vi "HFRR ADV v07.vi"() -> ()   [LabVIEW 2025] (continued)
            n1797 = local write "String 6"(w2052) -> ()
            n1798 = local write "String 7"(w2052) -> ()
            n1799 = local write "String 8"(w2052) -> ()
            n1800 = local write "String 12"(w2052) -> ()
            n1801 = local read "OK Button 16"() -> (w2037:bool)
            n1802 = String To Path(string=w2040) -> (path=w2048:path)
            n1803 = String To Path(string=w2039) -> (path=w2047:path)
            n1804 = String To Path(string=w2038) -> (path=w2046:path)
            n1805 = case shown="True" w2037 {
              tunnel: [w2053 w2054] -> w2041
              frame False {
                n1806 = local read "string1"() -> (w2053:string)
              }
              frame True {
                n1807 = local read "String Indicator 4"() -> (w2054:string)
              }
            }
            n1808 = Open/Create/Replace File "Open File"(file path (use dialog)=w2048) -> (refnum out=w2044:refnum<file>)  [unwired: 5 in, 2 out]
            n1809 = Open/Create/Replace File "Open File"(file path (use dialog)=w2047) -> (refnum out=w2043:refnum<file>)  [unwired: 5 in, 2 out]
            n1810 = Open/Create/Replace File "Open File"(file path (use dialog)=w2046) -> (refnum out=w2042:refnum<file>)  [unwired: 5 in, 2 out]
            n1811 = while {
              tunnel: w2044 -> [w2066]
              i -> [w2062]
              stop <- w2061 continue-if-true
              (unwired) TRUE ("line mode (F)")
              n1812 = Read from Text File "Read File"(file (use dialog)=w2066) -> (text=w2063:string)  [unwired: 3 in, 3 out]
              n1813 = local write "Numeric 11"(w2062) -> ()
              n1814 = String Length(string=w2063) -> (length=w2065:i32)
              n1815 = Greater?(x=w2065, y=1) -> (0:w2061:bool)
            }
            n1816 = while {
              tunnel: w2043 -> [w2072]
              i -> [w2068]
              stop <- w2067 continue-if-true
              (unwired) TRUE ("line mode (F)")
              n1817 = Read from Text File "Read File"(file (use dialog)=w2072) -> (text=w2069:string)  [unwired: 3 in, 3 out]
              n1818 = local write "Numeric 12"(w2068) -> ()
              n1819 = String Length(string=w2069) -> (length=w2071:i32)
              n1820 = Greater?(x=w2071, y=1) -> (0:w2067:bool)
            }
            n1821 = while {
              tunnel: w2042 -> [w2078]
              i -> [w2074]
              stop <- w2073 continue-if-true
              (unwired) TRUE ("line mode (F)")
              n1822 = Read from Text File "Read File"(file (use dialog)=w2078) -> (text=w2075:string)  [unwired: 3 in, 3 out]
              n1823 = local write "Numeric 13"(w2074) -> ()
              n1824 = String Length(string=w2075) -> (length=w2077:i32)
              n1825 = Greater?(x=w2077, y=1) -> (0:w2073:bool)
            }
            n1826 = String To Path(string=w2041) -> (path=w2049:path)
            n1827 = Open/Create/Replace File "Open File"(file path (use dialog)=w2049) -> (refnum out=w2045:refnum<file>)  [unwired: 5 in, 2 out]
            n1828 = while {
              tunnel: w2045 -> [w2060]
              i -> [w2056]
              stop <- w2055 continue-if-true
              (unwired) TRUE ("line mode (F)")
              n1829 = Read from Text File "Read File"(file (use dialog)=w2060) -> (text=w2057:string)  [unwired: 3 in, 3 out]
              n1830 = local write "Numeric 8"(w2056) -> ()
              n1831 = String Length(string=w2057) -> (length=w2059:i32)
              n1832 = Greater?(x=w2059, y=1) -> (0:w2055:bool)
            }
          }
          frame #1 {
            w2230 = FALSE ("ACTUAL   MERGE")
            # "Sample Temp"
            # "ECR"
            # "COF"
            # "Time\nCOF\nFF\nTemp"
            n1833 = case shown="True" w2103 {
              tunnel: [w2250 w2251] -> w2104
              frame False {
                n1834 = local read "string1"() -> (w2250:string)
              }
              frame True {
                n1835 = local read "String Indicator 4"() -> (w2251:string)
              }
            }
            n1836 = local read "string1 3"() -> (w2148:string)
            n1837 = String To Path(string=w2104) -> (path=w2235:path)
            n1838 = String To Path(string=w2148) -> (path=w2246:path)
            n1839 = local read "Numeric 12"() -> (w2232:i32)
            n1840 = local read "Numeric 8"() -> (w2234:i32)
            n1841 = local read "string1 2"() -> (w2149:string)
            n1842 = local read "string1 4"() -> (w2147:string)
            n1843 = Open/Create/Replace File "Open File"(file path (use dialog)=w2235) -> (refnum out=w2249:refnum<file>, error out=w2248:errorcluster)  [unwired: 5 in, 1 out]
            n1844 = Open/Create/Replace File "Open File"(file path (use dialog)=w2246) -> (refnum out=w2242:refnum<file>, error out=w2243:errorcluster)  [unwired: 5 in, 1 out]
            n1845 = for {
              N: w2234 -> [_]
              tunnel: w2249 -> [w2397]
              tunnel: w2248 -> [w2396]
              tunnel: [w2386] -> w2161 mode=indexing
              tunnel: [w2384] -> w2218 mode=indexing
              tunnel: [w2385] -> w2213 mode=indexing
              tunnel: w2230 -> [_]
              tunnel: [w2378] -> w2215 mode=indexing
              tunnel: [w2374] -> w2184 mode=indexing
              tunnel: [w2370] -> w2159 mode=indexing
              tunnel: [w2366] -> w2140 mode=indexing
              tunnel: [w2361] -> w2100 mode=indexing
              (unwired) TRUE ("line mode (F)")
              # "freq"
              # "Stroke"
              # "Time"
              # "CoF"
              # "Humidity"
              # "Temp"
              # "Air Temp"
              # "ECR"
              n1846 = Read from Text File "Read File"(file (use dialog)=w2397, error in=w2396) -> (text=w2362:string)  [unwired: 2 in, 3 out]
              n1847 = local write "String 6"(w2362) -> ()
              n1848 = String Subset(string=w2362, offset (0)=0, length (rest)=14 ("length (rest)")) -> (substring=w2390:string)
              n1849 = String Subset(string=w2362, offset (0)=35, length (rest)=9 ("length (rest)")) -> (substring=w2387:string)
              n1850 = String Subset(string=w2362, offset (0)=15, length (rest)=9 ("length (rest)")) -> (substring=w2393:string)
              n1851 = Fract/Exp String To Number(string=w2390) -> (number=w2386:dbl)  [unwired: 3 in, 1 out]
              n1852 = Fract/Exp String To Number(string=w2387) -> (number=w2385:dbl)  [unwired: 3 in, 1 out]
              n1853 = Fract/Exp String To Number(string=w2393) -> (number=w2384:dbl)  [unwired: 3 in, 1 out]
              n1854 = String Subset(string=w2362, offset (0)=85, length (rest)=9 ("length (rest)")) -> (substring=w2363:string)
              n1855 = String Subset(string=w2362, offset (0)=25, length (rest)=9 ("length (rest)")) -> (substring=w2369:string)
              n1856 = String Subset(string=w2362, offset (0)=55, length (rest)=9 ("length (rest)")) -> (substring=w2371:string)
              n1857 = String Subset(string=w2362, offset (0)=45, length (rest)=9 ("length (rest)")) -> (substring=w2377:string)
              n1858 = String Subset(string=w2362, offset (0)=65, length (rest)=9 ("length (rest)")) -> (substring=w2383:string)
              n1859 = Fract/Exp String To Number(string=w2369) -> (number=w2366:dbl)  [unwired: 3 in, 1 out]
              n1860 = Fract/Exp String To Number(string=w2363) -> (number=w2361:dbl)  [unwired: 3 in, 1 out]
              n1861 = Fract/Exp String To Number(string=w2371) -> (number=w2370:dbl)  [unwired: 3 in, 1 out]
              n1862 = Fract/Exp String To Number(string=w2377) -> (number=w2374:dbl)  [unwired: 3 in, 1 out]
              n1863 = Fract/Exp String To Number(string=w2383) -> (number=w2380:dbl)  [unwired: 3 in, 1 out]
              n1864 = Add(x=w2380, y=0.0) -> (x+y=w2378:dbl)
            }
            n1865 = for {
              N: w2232 -> [_]
              tunnel: w2243 -> [w2323]
              tunnel: w2242 -> [w2322]
              tunnel: [w2312] -> w2201 mode=indexing
              tunnel: [w2310] -> w2199 mode=indexing
              tunnel: [w2311] -> w2195 mode=indexing
              tunnel: w2230 -> [_]
              tunnel: [w2304] -> w2197 mode=indexing
              tunnel: [w2300] -> w2179 mode=indexing
              tunnel: [w2296] -> w2155 mode=indexing
              tunnel: [w2293] -> w2136 mode=indexing
              tunnel: [w2289] -> w2095 mode=indexing
              (unwired) 9 ("length (rest)")
              (unwired) 9 ("length (rest)")
              (unwired) TRUE ("line mode (F)")
              n1866 = Read from Text File "Read File"(file (use dialog)=w2322, error in=w2323) -> (text=w2290:string)  [unwired: 2 in, 3 out]
              n1867 = local write "String 8"(w2290) -> ()
              n1868 = String Subset(string=w2290, offset (0)=85) -> (substring=w2292:string)  [unwired: 1 in]
              n1869 = String Subset(string=w2290, offset (0)=35, length (rest)=9 ("length (rest)")) -> (substring=w2313:string)
              n1870 = String Subset(string=w2290, offset (0)=55, length (rest)=9 ("length (rest)")) -> (substring=w2298:string)
              n1871 = String Subset(string=w2290, offset (0)=25) -> (substring=w2294:string)  [unwired: 1 in]
              n1872 = String Subset(string=w2290, offset (0)=15, length (rest)=9 ("length (rest)")) -> (substring=w2319:string)
              n1873 = String Subset(string=w2290, offset (0)=0, length (rest)=14 ("length (rest)")) -> (substring=w2316:string)
              n1874 = String Subset(string=w2290, offset (0)=45, length (rest)=9 ("length (rest)")) -> (substring=w2303:string)
              n1875 = String Subset(string=w2290, offset (0)=65, length (rest)=9 ("length (rest)")) -> (substring=w2309:string)
              n1876 = Fract/Exp String To Number(string=w2292) -> (number=w2289:dbl)  [unwired: 3 in, 1 out]
              n1877 = Fract/Exp String To Number(string=w2313) -> (number=w2311:dbl)  [unwired: 3 in, 1 out]
              n1878 = Fract/Exp String To Number(string=w2298) -> (number=w2296:dbl)  [unwired: 3 in, 1 out]
              n1879 = Fract/Exp String To Number(string=w2294) -> (number=w2293:dbl)  [unwired: 3 in, 1 out]
              n1880 = Fract/Exp String To Number(string=w2319) -> (number=w2310:dbl)  [unwired: 3 in, 1 out]
              n1881 = Fract/Exp String To Number(string=w2316) -> (number=w2312:dbl)  [unwired: 3 in, 1 out]
              n1882 = Fract/Exp String To Number(string=w2303) -> (number=w2300:dbl)  [unwired: 3 in, 1 out]
              n1883 = Fract/Exp String To Number(string=w2309) -> (number=w2306:dbl)  [unwired: 3 in, 1 out]
              n1884 = Add(x=w2306, y=0.0) -> (x+y=w2304:dbl)
            }
            n1885 = String To Path(string=w2149) -> (path=w2247:path)
            n1886 = String To Path(string=w2147) -> (path=w2241:path)
            n1887 = local read "Numeric 11"() -> (w2231:i32)
            n1888 = local read "Numeric 13"() -> (w2233:i32)
            n1889 = Open/Create/Replace File "Open File"(file path (use dialog)=w2247) -> (refnum out=w2245:refnum<file>, error out=w2244:errorcluster)  [unwired: 5 in, 1 out]
            n1890 = Open/Create/Replace File "Open File"(file path (use dialog)=w2241) -> (refnum out=w2240:refnum<file>, error out=w2239:errorcluster)  [unwired: 5 in, 1 out]
            n1891 = for {
              N: w2231 -> [_]
              tunnel: w2245 -> [w2360]
              tunnel: w2244 -> [w2359]
              tunnel: [w2349] -> w2211 mode=indexing
              tunnel: [w2347] -> w2209 mode=indexing
              tunnel: [w2348] -> w2204 mode=indexing
              tunnel: w2230 -> [_]
              tunnel: [w2341] -> w2206 mode=indexing
              tunnel: [w2337] -> w2182 mode=indexing
              tunnel: [w2333] -> w2157 mode=indexing
              tunnel: [w2329] -> w2138 mode=indexing
              tunnel: [w2324] -> w2096 mode=indexing
              (unwired) TRUE ("line mode (F)")
              n1892 = Read from Text File "Read File"(file (use dialog)=w2360, error in=w2359) -> (text=w2325:string)  [unwired: 2 in, 3 out]
              n1893 = local write "String 7"(w2325) -> ()
              n1894 = String Subset(string=w2325, offset (0)=85, length (rest)=9 ("length (rest)")) -> (substring=w2328:string)
              n1895 = String Subset(string=w2325, offset (0)=35, length (rest)=9 ("length (rest)")) -> (substring=w2350:string)
              n1896 = String Subset(string=w2325, offset (0)=55, length (rest)=9 ("length (rest)")) -> (substring=w2336:string)
              n1897 = String Subset(string=w2325, offset (0)=25, length (rest)=9 ("length (rest)")) -> (substring=w2330:string)
              n1898 = String Subset(string=w2325, offset (0)=45, length (rest)=9 ("length (rest)")) -> (substring=w2338:string)
              n1899 = String Subset(string=w2325, offset (0)=0, length (rest)=14 ("length (rest)")) -> (substring=w2353:string)
              n1900 = String Subset(string=w2325, offset (0)=15, length (rest)=9 ("length (rest)")) -> (substring=w2356:string)
              n1901 = String Subset(string=w2325, offset (0)=65, length (rest)=9 ("length (rest)")) -> (substring=w2342:string)
              n1902 = Fract/Exp String To Number(string=w2328) -> (number=w2324:dbl)  [unwired: 3 in, 1 out]
              n1903 = Fract/Exp String To Number(string=w2350) -> (number=w2348:dbl)  [unwired: 3 in, 1 out]
              n1904 = Fract/Exp String To Number(string=w2336) -> (number=w2333:dbl)  [unwired: 3 in, 1 out]
              n1905 = Fract/Exp String To Number(string=w2330) -> (number=w2329:dbl)  [unwired: 3 in, 1 out]
              n1906 = Fract/Exp String To Number(string=w2338) -> (number=w2337:dbl)  [unwired: 3 in, 1 out]
              n1907 = Fract/Exp String To Number(string=w2353) -> (number=w2349:dbl)  [unwired: 3 in, 1 out]
              n1908 = Fract/Exp String To Number(string=w2356) -> (number=w2347:dbl)  [unwired: 3 in, 1 out]
              n1909 = Fract/Exp String To Number(string=w2342) -> (number=w2345:dbl)  [unwired: 3 in, 1 out]
              n1910 = Add(x=w2345, y=0.0) -> (x+y=w2341:dbl)
            }
            n1911 = for {
              N: w2233 -> [_]
              tunnel: w2240 -> [w2288]
              tunnel: w2239 -> [w2287]
              tunnel: [w2277] -> w2193 mode=indexing
              tunnel: [w2276] -> w2186 mode=indexing
              tunnel: w2230 -> [_]
              tunnel: [w2265] -> w2191 mode=indexing
              tunnel: [w2270] -> w2188 mode=indexing
              tunnel: [w2266] -> w2178 mode=indexing
              tunnel: [w2261] -> w2153 mode=indexing
              tunnel: [w2257] -> w2134 mode=indexing
              tunnel: [w2252] -> w2094 mode=indexing
              (unwired) 1.0 ("x")
              (unwired) TRUE ("line mode (F)")
              n1912 = Read from Text File "Read File"(file (use dialog)=w2288, error in=w2287) -> (text=w2253:string)  [unwired: 2 in, 3 out]
              n1913 = local write "String 12"(w2253) -> ()
              n1914 = String Subset(string=w2253, offset (0)=85, length (rest)=9 ("length (rest)")) -> (substring=w2255:string)
              n1915 = String Subset(string=w2253, offset (0)=35, length (rest)=9 ("length (rest)")) -> (substring=w2278:string)
              n1916 = String Subset(string=w2253, offset (0)=55, length (rest)=9 ("length (rest)")) -> (substring=w2263:string)
              n1917 = String Subset(string=w2253, offset (0)=25, length (rest)=9 ("length (rest)")) -> (substring=w2259:string)
              n1918 = String Subset(string=w2253, offset (0)=45, length (rest)=9 ("length (rest)")) -> (substring=w2268:string)
              n1919 = String Subset(string=w2253, offset (0)=15, length (rest)=9 ("length (rest)")) -> (substring=w2284:string)
              n1920 = String Subset(string=w2253, offset (0)=0, length (rest)=14 ("length (rest)")) -> (substring=w2281:string)
              n1921 = String Subset(string=w2253, offset (0)=65, length (rest)=9 ("length (rest)")) -> (substring=w2271:string)
              n1922 = Fract/Exp String To Number(string=w2255) -> (number=w2252:dbl)  [unwired: 3 in, 1 out]
              n1923 = Fract/Exp String To Number(string=w2278) -> (number=w2276:dbl)  [unwired: 3 in, 1 out]
              n1924 = Fract/Exp String To Number(string=w2263) -> (number=w2261:dbl)  [unwired: 3 in, 1 out]
              n1925 = Fract/Exp String To Number(string=w2259) -> (number=w2257:dbl)  [unwired: 3 in, 1 out]
              n1926 = Fract/Exp String To Number(string=w2268) -> (number=w2266:dbl)  [unwired: 3 in, 1 out]
              n1927 = Fract/Exp String To Number(string=w2284) -> (number=w2265:dbl)  [unwired: 3 in, 1 out]
              n1928 = Fract/Exp String To Number(string=w2281) -> (number=w2277:dbl)  [unwired: 3 in, 1 out]
              n1929 = Fract/Exp String To Number(string=w2271) -> (number=w2274:dbl)  [unwired: 3 in, 1 out]
              n1930 = Add(x=w2274, y=0.0) -> (x+y=w2270:dbl)
            }
            n1931 = Delete From Array(array=w2136, index=0) -> (array with subset deleted=w2109:dbl[])  [unwired: 1 in, 1 out]
            n1932 = Delete From Array(array=w2199, index=0) -> (array with subset deleted=w2172:dbl[])  [unwired: 1 in, 1 out]
            n1933 = Delete From Array(array=w2179, index=0) -> (array with subset deleted=w2167:dbl[])  [unwired: 1 in, 1 out]
            n1934 = Delete From Array(array=w2197, index=0) -> (array with subset deleted=w2198:dbl[])  [unwired: 1 in, 1 out]
            n1935 = call-poly <vilib>:"Mean.vi"("X"=w2109) -> ("mean"=→"КОФ2 4":dbl)  [unwired: 1 out]
            n1936 = call-poly <vilib>:"Mean.vi"("X"=w2172) -> ("mean"=→"КОФ3":dbl)  [unwired: 1 out]
            n1937 = call-poly <vilib>:"Mean.vi"("X"=w2167) -> ("mean"=→"CP3":dbl)  [unwired: 1 out]
            n1938 = Delete From Array(array=w2161, index=0) -> (array with subset deleted=w2088:dbl[])  [unwired: 1 in, 1 out]
            n1939 = Delete From Array(array=w2100, index=0) -> (array with subset deleted=w2087:dbl[])  [unwired: 1 in, 1 out]
            n1940 = Delete From Array(array=w2140, index=0) -> (array with subset deleted=w2111:dbl[])  [unwired: 1 in, 1 out]
            n1941 = Delete From Array(array=w2218, index=0) -> (array with subset deleted=w2173:dbl[])  [unwired: 1 in, 1 out]
            n1942 = Delete From Array(array=w2184, index=0) -> (array with subset deleted=w2169:dbl[])  [unwired: 1 in, 1 out]
            "array w/ subset deleted" <- w2169
            n1943 = Delete From Array(array=w2215, index=0) -> (array with subset deleted=w2216:dbl[])  [unwired: 1 in, 1 out]
            n1944 = call-poly <vilib>:"Mean.vi"("X"=w2111) -> ("mean"=→"КОФ2 2":dbl)  [unwired: 1 out]
            n1945 = call-poly <vilib>:"Mean.vi"("X"=w2173) -> ("mean"=→"КОФ1":dbl)  [unwired: 1 out]
            n1946 = Bundle "Bundle"(w2088, w2087) -> (w2093:cluster{dbl[], dbl[]})  [unwired: 1 in]
            n1947 = Bundle "Bundle"(w2088, w2216) -> (w2080:cluster{dbl[], dbl[]})  [unwired: 1 in]
            n1948 = Delete From Array(array=w2095, index=0) -> (array with subset deleted=w2083:dbl[])  [unwired: 1 in, 1 out]
            n1949 = Delete From Array(array=w2096, index=0) -> (array with subset deleted=w2085:dbl[])  [unwired: 1 in, 1 out]
            n1950 = Delete From Array(array=w2206, index=0) -> (array with subset deleted=w2207:dbl[])  [unwired: 1 in, 1 out]
            n1951 = Delete From Array(array=w2094, index=0) -> (array with subset deleted=w2081:dbl[])  [unwired: 1 in, 1 out]
            n1952 = Delete From Array(array=w2188, index=0) -> (array with subset deleted=w2189:dbl[])  [unwired: 1 in, 1 out]
            n1953 = Delete From Array(array=w2213, index=0) -> (array with subset deleted=w2119:dbl[])  [unwired: 1 in, 1 out]
            n1954 = Delete From Array(array=w2159, index=0) -> (array with subset deleted=w2115:dbl[])  [unwired: 1 in, 1 out]
            n1955 = Delete From Array(array=w2195, index=0) -> (array with subset deleted=w2117:dbl[])  [unwired: 1 in, 1 out]
            n1956 = Delete From Array(array=w2155, index=0) -> (array with subset deleted=w2113:dbl[])  [unwired: 1 in, 1 out]
            n1957 = Delete From Array(array=w2204, index=0) -> (array with subset deleted=w2118:dbl[])  [unwired: 1 in, 1 out]
            n1958 = Delete From Array(array=w2157, index=0) -> (array with subset deleted=w2114:dbl[])  [unwired: 1 in, 1 out]
            n1959 = Delete From Array(array=w2138, index=0) -> (array with subset deleted=w2110:dbl[])  [unwired: 1 in, 1 out]
            n1960 = Delete From Array(array=w2182, index=0) -> (array with subset deleted=w2168:dbl[])  [unwired: 1 in, 1 out]
            n1961 = Delete From Array(array=w2209, index=0) -> (array with subset deleted=w2170:dbl[])  [unwired: 1 in, 1 out]
            n1962 = Delete From Array(array=w2186, index=0) -> (array with subset deleted=w2116:dbl[])  [unwired: 1 in, 1 out]
            n1963 = Delete From Array(array=w2153, index=0) -> (array with subset deleted=w2112:dbl[])  [unwired: 1 in, 1 out]
            n1964 = Delete From Array(array=w2134, index=0) -> (array with subset deleted=w2108:dbl[])  [unwired: 1 in, 1 out]
            n1965 = Delete From Array(array=w2178, index=0) -> (array with subset deleted=w2166:dbl[])  [unwired: 1 in, 1 out]
            n1966 = Delete From Array(array=w2191, index=0) -> (array with subset deleted=w2171:dbl[])  [unwired: 1 in, 1 out]
            n1967 = Delete From Array(array=w2201, index=0) -> (array with subset deleted=w2084:dbl[])  [unwired: 1 in, 1 out]
            n1968 = Delete From Array(array=w2211, index=0) -> (array with subset deleted=w2086:dbl[])  [unwired: 1 in, 1 out]
            n1969 = Delete From Array(array=w2193, index=0) -> (array with subset deleted=w2082:dbl[])  [unwired: 1 in, 1 out]
            n1970 = Bundle "Bundle"(w2088, w2119) -> (w2106:cluster{dbl[], dbl[]})  [unwired: 1 in]
            n1971 = Bundle "Bundle"(w2088, w2173) -> (w2107:cluster{dbl[], dbl[]})  [unwired: 1 in]
            n1972 = Bundle "Bundle"(w2119, w2115) -> (w2121:cluster{dbl[], dbl[]})  [unwired: 1 in]
            n1973 = Bundle "Bundle"(w2084, w2083) -> (w2091:cluster{dbl[], dbl[]})  [unwired: 1 in]
            n1974 = Bundle "Bundle"(w2117, w2113) -> (w2123:cluster{dbl[], dbl[]})  [unwired: 1 in]
            n1975 = Bundle "Bundle"(w2084, w2117) -> (w2227:cluster{dbl[], dbl[]})  [unwired: 1 in]
            n1976 = Bundle "Bundle"(w2084, w2113) -> (w2151:cluster{dbl[], dbl[]})  [unwired: 1 in]
            n1977 = Bundle "Bundle"(w2084, w2172) -> (w2237:cluster{dbl[], dbl[]})  [unwired: 1 in]
            n1978 = Bundle "Bundle"(w2084, w2167) -> (w2175:cluster{dbl[], dbl[]})  [unwired: 1 in]
            n1979 = Bundle "Bundle"(w2084, w2198) -> (w2222:cluster{dbl[], dbl[]})  [unwired: 1 in]
            n1980 = Bundle "Bundle"(w2118, w2114) -> (w2122:cluster{dbl[], dbl[]})  [unwired: 1 in]
            n1981 = Bundle "Bundle"(w2086, w2085) -> (w2092:cluster{dbl[], dbl[]})  [unwired: 1 in]
            n1982 = Bundle "Bundle"(w2086, w2118) -> (w2229:cluster{dbl[], dbl[]})  [unwired: 1 in]
            n1983 = Bundle "Bundle"(w2086, w2114) -> (w2152:cluster{dbl[], dbl[]})  [unwired: 1 in]
            n1984 = Bundle "Bundle"(w2086, w2168) -> (w2176:cluster{dbl[], dbl[]})  [unwired: 1 in]
            n1985 = Bundle "Bundle"(w2086, w2170) -> (w2238:cluster{dbl[], dbl[]})  [unwired: 1 in]
            n1986 = Bundle "Bundle"(w2086, w2207) -> (w2220:cluster{dbl[], dbl[]})  [unwired: 1 in]
            n1987 = Bundle "Bundle"(w2116, w2112) -> (w2124:cluster{dbl[], dbl[]})  [unwired: 1 in]
            n1988 = Bundle "Bundle"(w2082, w2081) -> (w2090:cluster{dbl[], dbl[]})  [unwired: 1 in]
            n1989 = Bundle "Bundle"(w2082, w2116) -> (w2228:cluster{dbl[], dbl[]})  [unwired: 1 in]
            n1990 = Bundle "Bundle"(w2082, w2112) -> (w2150:cluster{dbl[], dbl[]})  [unwired: 1 in]
            n1991 = Bundle "Bundle"(w2082, w2166) -> (w2174:cluster{dbl[], dbl[]})  [unwired: 1 in]
            n1992 = Bundle "Bundle"(w2082, w2171) -> (w2236:cluster{dbl[], dbl[]})  [unwired: 1 in]
            n1993 = Bundle "Bundle"(w2082, w2189) -> (w2221:cluster{dbl[], dbl[]})  [unwired: 1 in]
            n1994 = call-poly <vilib>:"Mean.vi"("X"=w2169) -> ("mean"=→"CP1":dbl)  [unwired: 1 out]
            n1995 = call-poly <vilib>:"Mean.vi"("X"=w2110) -> ("mean"=→"КОФ2 3":dbl)  [unwired: 1 out]
            n1996 = call-poly <vilib>:"Mean.vi"("X"=w2168) -> ("mean"=→"CP2":dbl)  [unwired: 1 out]
            n1997 = call-poly <vilib>:"Mean.vi"("X"=w2170) -> ("mean"=→"КОФ2":dbl)  [unwired: 1 out]
            n1998 = call-poly <vilib>:"Mean.vi"("X"=w2108) -> ("mean"=→"КОФ2 5":dbl)  [unwired: 1 out]
            n1999 = call-poly <vilib>:"Mean.vi"("X"=w2166) -> ("mean"=→"CP4":dbl)  [unwired: 1 out]
            n2000 = call-poly <vilib>:"Mean.vi"("X"=w2171) -> ("mean"=→"КОФ4":dbl)  [unwired: 1 out]
            n2001 = Bundle "Bundle"(w2088, w2115) -> (w2079:cluster{dbl[], dbl[]})  [unwired: 1 in]
            n2002 = Bundle "Bundle"(w2088, w2169) -> (w2102:cluster{dbl[], dbl[]})  [unwired: 1 in]
            n2003 = Build Array "Build Array"(w2079, w2102) -> (w2105:cluster{dbl[], dbl[]}[])
            "XY Graph 17" <- w2105
            n2004 = Build Array "Build Array"(w2093, w2092, w2091, w2090) -> (→"Frequency ( Hz )":cluster{dbl[], dbl[]}[])
            n2005 = Build Array "Build Array"(w2121, w2122, w2123, w2124) -> (→"Air Temp ( °C ) vs Humidity ( % RH )":cluster{dbl[], dbl[]}[])
            n2006 = Build Array "Build Array"(w2106, w2229, w2227, w2228) -> (→"Air Temperature  ( °C )":cluster{dbl[], dbl[]}[])
            n2007 = Build Array "Build Array"(w2079, w2152, w2151, w2150) -> (→"Humidity ( %RH )":cluster{dbl[], dbl[]}[])
            n2008 = Build Array "Build Array"(w2107, w2238, w2237, w2236) -> (→"Coefficient Of Friction":cluster{dbl[], dbl[]}[])
            n2009 = Build Array "Build Array"(w2102, w2176, w2175, w2174) -> (→"Sample Temperature ( °C )":cluster{dbl[], dbl[]}[])
            n2010 = Build Array "Build Array"(w2080, w2220, w2222, w2221) -> (→"XY Graph 13":cluster{dbl[], dbl[]}[])
            n2011 = Bundle "Bundle"(w2088, w2111) -> (w2133:cluster{dbl[], dbl[]})  [unwired: 1 in]
            n2012 = Bundle "Bundle"(w2084, w2109) -> (w2131:cluster{dbl[], dbl[]})  [unwired: 1 in]
            n2013 = Bundle "Bundle"(w2086, w2110) -> (w2132:cluster{dbl[], dbl[]})  [unwired: 1 in]
            n2014 = Bundle "Bundle"(w2082, w2108) -> (w2130:cluster{dbl[], dbl[]})  [unwired: 1 in]
            n2015 = Build Array "Build Array"(w2133, w2132, w2131, w2130) -> (→"Stroke ( mm )":cluster{dbl[], dbl[]}[])
            n2016 = local write "XY Graph 16"(w2105) -> ()
          }
          frame #2 {
          }
          frame #3 {
            n2017 = local write "Numeric 8"(0 ("Numeric 8")) -> ()
            n2018 = local write "Numeric 11"(0 ("Numeric 11")) -> ()
            n2019 = local write "Numeric 12"(0 ("Numeric 12")) -> ()
            n2020 = local write "Numeric 13"(0 ("Numeric 13")) -> ()
            n2021 = property on="OPEN" class="Bool (strict)"("Visible"=TRUE) -> ()  [unwired: 2 in, 2 out]
            n2022 = local read "String Control 2"() -> (w2405:string)
            n2023 = local read "String Control 4"() -> (w2404:string)
            n2024 = local read "String Control 6"() -> (w2403:string)
            n2025 = local read "String Control 8"() -> (w2402:string)
            n2026 = Match Pattern(string=w2405, regular expression="Samples / cycle :- ") -> (after substring=w2419:string)  [unwired: 1 in, 3 out]
            n2027 = Match Pattern(string=w2405, regular expression="Frequency :- ") -> (after substring=w2438:string)  [unwired: 1 in, 3 out]
            n2028 = Match Pattern(string=w2404, regular expression="Samples / cycle :- ") -> (after substring=w2415:string)  [unwired: 1 in, 3 out]
            n2029 = Match Pattern(string=w2404, regular expression="Frequency :- ") -> (after substring=w2433:string)  [unwired: 1 in, 3 out]
            n2030 = Match Pattern(string=w2403, regular expression="Samples / cycle :- ") -> (after substring=w2411:string)  [unwired: 1 in, 3 out]
            n2031 = Match Pattern(string=w2403, regular expression="Frequency :- ") -> (after substring=w2428:string)  [unwired: 1 in, 3 out]
            n2032 = Match Pattern(string=w2402, regular expression="Samples / cycle :- ") -> (after substring=w2407:string)  [unwired: 1 in, 3 out]
            n2033 = Match Pattern(string=w2402, regular expression="Frequency :- ") -> (after substring=w2423:string)  [unwired: 1 in, 3 out]
            n2034 = String Subset(string=w2419, length (rest)=6 ("length (rest)")) -> (substring=w2421:string)  [unwired: 1 in]
            n2035 = String Subset(string=w2438, length (rest)=9 ("length (rest)")) -> (substring=w2440:string)  [unwired: 1 in]
            n2036 = String Subset(string=w2415, length (rest)=6 ("length (rest)")) -> (substring=w2417:string)  [unwired: 1 in]
            n2037 = String Subset(string=w2433, length (rest)=9 ("length (rest)")) -> (substring=w2435:string)  [unwired: 1 in]
            n2038 = String Subset(string=w2411, length (rest)=6 ("length (rest)")) -> (substring=w2413:string)  [unwired: 1 in]
            n2039 = String Subset(string=w2428, length (rest)=9 ("length (rest)")) -> (substring=w2430:string)  [unwired: 1 in]
            n2040 = String Subset(string=w2407, length (rest)=6 ("length (rest)")) -> (substring=w2409:string)  [unwired: 1 in]
            n2041 = String Subset(string=w2423, length (rest)=9 ("length (rest)")) -> (substring=w2425:string)  [unwired: 1 in]
            n2042 = Fract/Exp String To Number(string=w2421) -> (number=w2401:dbl)  [unwired: 3 in, 1 out]
            n2043 = Fract/Exp String To Number(string=w2440) -> (number=w2441:dbl)  [unwired: 3 in, 1 out]
            n2044 = Fract/Exp String To Number(string=w2417) -> (number=w2400:dbl)  [unwired: 3 in, 1 out]
            n2045 = Fract/Exp String To Number(string=w2435) -> (number=w2436:dbl)  [unwired: 3 in, 1 out]
            n2046 = Fract/Exp String To Number(string=w2413) -> (number=w2399:dbl)  [unwired: 3 in, 1 out]
            n2047 = Fract/Exp String To Number(string=w2430) -> (number=w2431:dbl)  [unwired: 3 in, 1 out]
            n2048 = Fract/Exp String To Number(string=w2409) -> (number=w2398:dbl)  [unwired: 3 in, 1 out]
            n2049 = Fract/Exp String To Number(string=w2425) -> (number=w2426:dbl)  [unwired: 3 in, 1 out]
            n2050 = local write "sample1"(w2401) -> ()
            n2051 = local write "freq1"(w2441) -> ()
            n2052 = local write "sample2"(w2400) -> ()
            n2053 = local write "freq2"(w2436) -> ()
            n2054 = local write "sample3"(w2399) -> ()
            n2055 = local write "freq3"(w2431) -> ()
            n2056 = local write "sample4"(w2398) -> ()
            n2057 = local write "freq 4"(w2426) -> ()
          }
        }
      }
    }
    n2058 = case shown="True" w1889 {
      selector: w1889 -> [_ w2018]
      frame False {
      }
      frame True {
        n2059 = Not(x=w2018) -> (.not. x?=w2014:bool)
        n2060 = local write "service 3"(w2014) -> ()
        n2061 = local write "OPEN 6"(w2014) -> ()
        n2062 = call <vilib>:"System Exec.vi"("wait until completion? (T)"=TRUE, "command line"="C:\\LAB-IQ\\Scar View.exe") -> ("error out"=→"error out 5":errorcluster)  [unwired: 6 in, 3 out]
      }
    }
    n2063 = case shown="\"Acquire\", Default" w1901 {
      frame "Acquire", Default {
        w2922 = 0.2 ("y")
        w2927 = 1.0 ("y")
        w2928 = 0.8 ("y")
        # "Elapsed time\ncof\nstroke\nAir temp\nTemp\nHumidity"
        n2064 = disable-structure shown="Disabled" {
          frame Disabled {
            n2065 = local read "Flag"() -> (w2945:dbl)
            n2066 = local read "RUN"() -> (w2942:bool)
            n2067 = Not(x=w2942) -> (.not. x?=w2941:bool)
            n2068 = Equal?(x=w2945, y=10.0) -> (x = y?=w2943:bool)
            n2069 = And(x=w2943, y=w2941) -> (x .and. y?=w2940:bool)
            n2070 = case shown="True" w2940 {
              frame False {
              }
              frame True {
                w2946 = FALSE ("Heater Button")
                n2071 = local write "Humidity"(w2946) -> ()
                n2072 = local write "Heater Button"(w2946) -> ()
              }
            }
          }
          frame Enabled {
          }
        }
        n2073 = disable-structure shown="Disabled" {
          frame Disabled {
            n2074 = case shown="True" {
              selector: _ -> [_ _]
              frame False {
              }
              frame True {
                w3037 = TRUE ("Heater")
                n2075 = local write "Humidity"(w3037) -> ()
                n2076 = local write "Heater Button"(w3037) -> ()
                n2077 = local read "TEST STANDARD"() -> (w3040:T4)
                n2078 = local read "TEST STANDARD"() -> (w3035:T4)
                n2079 = Equal?(x=w3040, y=enum16{"ASTM D6079", "ISO 12156", "Custom"}."ISO 12156" ("Test Standard")) -> (x = y?=w3038:bool)
                n2080 = Equal?(x=w3035, y=enum16{"ASTM D6079", "ISO 12156", "Custom"}."ASTM D6079" ("Test Standard")) -> (x = y?=w3034:bool)
                n2081 = case shown="True" w3038 {
                  frame False {
                  }
                  frame True {
                    n2082 = local write "Heater"(TRUE ("Heater")) -> ()
                    n2083 = local write "airtempflg"(FALSE ("airtempflg")) -> ()
                  }
                }
                n2084 = case shown="True" w3034 {
                  frame False {
                  }
                  frame True {
                    n2085 = local write "Heater"(FALSE ("Heater")) -> ()
                    n2086 = local write "airtempflg"(TRUE ("airtempflg")) -> ()
                  }
                }
              }
            }
          }
          frame Enabled {
          }
        }
        n2087 = stacked-sequence {
          frame #0 {
            n2088 = case shown="True" "RST FF" {
              frame False {
              }
              frame True {
                w3103 = 0.0 ("X Scale.Range:Maximum")
                n2089 = property on="Frictional Force ( N )" class="WFChart (strict)"("XScale.Maximum"=600.0 ("X Scale.Range:Maximum"), "XScale.Minimum"=w3103, "YScale.Maximum"=10.0 ("Y Scale.Range:Maximum"), "YScale.Minimum"=w3103) -> ()  [unwired: 2 in, 2 out]
              }
            }
          }
          frame #1 {
            n2090 = case shown="True" "RST TEMP" {
              frame False {
              }
              frame True {
                n2091 = property on="Temperature ( Deg C )" class="WFChart (strict)"("XScale.Minimum"=0.0 ("X Scale.Range:Minimum"), "XScale.Maximum"=600.0 ("X Scale.Range:Maximum"), "YScale.Minimum"=0.0 ("Y Scale.Range:Minimum"), "YScale.Maximum"=100.0 ("Y Scale.Range:Maximum")) -> ()  [unwired: 2 in, 2 out]
              }
            }
          }
          frame #2 {
            n2092 = case shown="True" "RSTCOF" {
              frame False {
              }
              frame True {
                n2093 = property on="Coefficient of Friction" class="WFChart (strict)"("XScale.Minimum"=0.0 ("X Scale.Range:Minimum"), "XScale.Maximum"=600.0 ("X Scale.Range:Maximum"), "YScale.Maximum"=1.0 ("X Scale.Range:Minimum"), "YScale.Minimum"=0.0 ("X Scale.Range:Minimum")) -> ()  [unwired: 2 in, 2 out]
              }
            }
          }
          frame #3 {
            n2094 = case shown="True" "RSTCOF 2" {
              frame False {
              }
              frame True {
                (unwired) 100.0 ("Y Scale.Range:Maximum")
                (unwired) 0.0 ("Y Scale.Range:Minimum")
                (unwired) 600.0 ("X Scale.Range:Maximum")
                (unwired) 0.0 ("X Scale.Range:Minimum")
              }
            }
          }
          frame #4 {
            n2095 = case shown="True" "RSTCOF 3" {
              frame False {
              }
              frame True {
                n2096 = property on="Electrical Contact Resistance ( % )" class="WFChart (strict)"("XScale.Minimum"=0.0 ("X Scale.Range:Minimum"), "XScale.Maximum"=600.0 ("X Scale.Range:Maximum"), "YScale.Minimum"=0.0 ("Y Scale.Range:Minimum"), "YScale.Maximum"=100.0 ("Y Scale.Range:Maximum")) -> ()  [unwired: 2 in, 2 out]
              }
            }
          }
        }
        n2097 = disable-structure shown="Disabled" {
          frame Disabled {
            n2098 = case shown="True" {
              selector: _ -> [_ _]
              frame False {
              }
              frame True {
                n2099 = local read "zflag 2"() -> (w3004:dbl)
                n2100 = local read "yflag"() -> (w3006:dbl)
                n2101 = Equal?(x=w3006, y=2.0 ("tflag")) -> (x = y?=w3008:bool)
                n2102 = Equal?(x=w3004, y=3.0 ("tflag")) -> (x = y?=w3007:bool)
                n2103 = And(x=w3008, y=w3007) -> (x .and. y?=w3002:bool)
                n2104 = case shown="True" w3002 {
                  frame False {
                  }
                  frame True {
                    w3033 = 0.0 ("zflag")
                    n2105 = local write "zflag"(w3033) -> ()
                    n2106 = local write "zflag 2"(w3033) -> ()
                    n2107 = Delete(path (use dialog)=path "C:/LAB-IQ-NXT/WO 2449 TT.sig" ("file path (dialog if empty)")) -> (deleted path=w3032:path)  [unwired: 4 in, 2 out]
                    n2108 = Delete(path (use dialog)=path "C:/LAB-IQ-NXT/WO 2449 TRH.sig" ("file path (dialog if empty)")) -> (deleted path=w3027:path)  [unwired: 4 in, 2 out]
                    n2109 = local read "SEN.RUN HRS"() -> (w3019:dbl)
                    n2110 = local read "SENSOR TIME"() -> (w3017:dbl)
                    n2111 = call <vilib>:"compatOverwrite.vi"("overwrite (F)"=TRUE) -> ("overwrite?"=w3009:T22)
                    n2112 = call <vilib>:"compatOverwrite.vi"("overwrite (F)"=TRUE) -> ("overwrite?"=w3013:T22)
                    n2113 = local read "Total No. of Tests"() -> (w3020:dbl)
                    n2114 = Add(x=w3017, y=w3019) -> (x+y=w3018:dbl)
                    "SEN.RUN HRS" <- w3018
                    n2115 = Open/Create/Replace File(file path (use dialog)=w3032, operation (0:open)=w3009) -> (refnum out=w3010:refnum<file>, error out=w3011:errorcluster)  [unwired: 4 in, 1 out]
                    n2116 = Open/Create/Replace File(file path (use dialog)=w3027, operation (0:open)=w3013) -> (refnum out=w3014:refnum<file>, error out=w3015:errorcluster)  [unwired: 4 in, 1 out]
                    n2117 = Deny Access(4:w3011, 6:T20."deny none" ("deny mode (2)"), 7:w3010) -> (3:w3031:refnum<file>)  [unwired: 1 out]
                    n2118 = Deny Access(4:w3015, 6:T20."deny none" ("deny mode (2)"), 7:w3014) -> (3:w3023:refnum<file>)  [unwired: 1 out]
                    n2119 = Number To Decimal String(number=w3020) -> (decimal integer string=w3028:string)  [unwired: 1 in]
                    n2120 = Number To Decimal String(number=w3018) -> (decimal integer string=w3024:string)  [unwired: 1 in]
                    n2121 = Write to Binary File(file (use dialog)=w3031, data=w3028, 5:FALSE ("prepend array or string size? (T)")) -> ()  [unwired: 3 in, 3 out]
                    n2122 = Write to Binary File(file (use dialog)=w3023, data=w3024, 5:FALSE ("prepend array or string size? (T)")) -> ()  [unwired: 3 in, 3 out]
                  }
                }
              }
            }
          }
          frame Enabled {
          }
        }
        n2123 = local read "RUN"() -> (w2931:bool)
        n2124 = local read "run replace"() -> (w2935:bool)
        n2125 = local read "run replace"() -> (w2934:bool)
        n2126 = case shown="True" w2931 {
          frame False {
            n2127 = local write "run replace"(FALSE ("run replace")) -> ()
          }
          frame True {
            "run replace" <- TRUE ("run replace")
          }
        }
        n2128 = local read "RUN"() -> (w2939:bool)
        n2129 = local read "Set Temp"() -> (w2901:dbl)
        n2130 = local read "SetTemp"() -> (w2903:dbl)
        n2131 = case shown="False" w2939 {
          tunnel: [FALSE ("TEST RUNNING") TRUE ("TEST RUNNING")] -> w2938
          frame False {
            w3122 = 0.0 ("Flag")
            n2132 = local write "Elapsed time"(0.0 ("elapsedtime")) -> ()
            n2133 = local write "Time Remaining"(w3122) -> ()
            n2134 = local write "Flag"(w3122) -> ()
          }
          frame True {
            n2135 = local write "Flag"(10.0 ("Flag")) -> ()
          }
        }
        n2136 = case shown="False" w2935 {
          frame False {
            n2137 = local read "zflag"() -> (→"zflag 2":dbl)
            n2138 = local write "yflag"(2.0 ("tflag")) -> ()
            n2139 = local write "FLAG 4"(0.0 ("FLAG")) -> ()
          }
          frame True {
            n2140 = local write "yflag"(1.0 ("tflag")) -> ()
            n2141 = local write "zflag"(3.0 ("zflag")) -> ()
          }
        }
        n2142 = local read "acq 2"() -> (w2933:bool)
        n2143 = local read "AIR TEMP"() -> (w2896:dbl)
        n2144 = local read "Amb temp"() -> (w2900:dbl)
        n2145 = case shown="True" "Save & Continue" {
          frame False {
          }
          frame True {
            "acq 2" <- TRUE ("acq 2")
          }
        }
        n2146 = local read "Set Rh"() -> (w2902:dbl)
        n2147 = Add(x=w2903, y=w2928) -> (x+y=w2929:dbl)
        n2148 = Subtract(x=w2903, y=w2928) -> (x-y=w2930:dbl)
        n2149 = Add(x=w2901, y=w2922) -> (x+y=w2923:dbl)
        n2150 = Subtract(x=w2901, y=w2922) -> (x-y=w2924:dbl)
        n2151 = And(x=w2933, y=w2934) -> (x .and. y?=w2932:bool)
        n2152 = Greater Or Equal?(x=w2896, y=15.0) -> (x >= y?=w2897:bool)
        "powstat" <- w2897
        n2153 = local read "Humidity ( %RH )"() -> (w2899:dbl)
        n2154 = case shown="True" "Save & Continue" {
          frame False {
          }
          frame True {
            n2155 = while {
              tunnel: "0123456789abcdefghijklmnopqrstuvwxyzABCDEFGHIJKLMNOPQRSTUVWXYZ" ("string 2") -> [w3093]
              shift-right: [w3091] -> w3086
              shift-left: "" -> [w3090]
              i -> [w3100]
              stop <- w3099 stop-if-true
              n2156 = Random Number (0-1)() -> (number: 0 to 1=w3094:dbl)
              n2157 = Multiply(x=w3094, y=62.0) -> (x*y=w3096:dbl)
              n2158 = Decrement(x="Length") -> (x-1=w3089:i16)
              n2159 = To Word Integer(number=w3096) -> (16bit integer=w3097:i16)
              n2160 = String Subset(string=w3093, offset (0)=w3097, length (rest)=1 ("length (rest)")) -> (substring=w3092:string)
              n2161 = Greater Or Equal?(x=w3100, y=w3089) -> (x >= y?=w3099:bool)
              n2162 = Concatenate Strings(w3092, w3090) -> (w3091:string)
            }
            n2163 = local write "UUID"(w3086) -> ()
          }
        }
        n2164 = In Range and Coerce(upper limit=w2929, x=w2900, lower limit=w2930) -> (In Range?=w2919:bool)  [unwired: 1 out]
        n2165 = Add(x=w2902, y=w2927) -> (x+y=w2926:dbl)
        n2166 = Subtract(x=w2902, y=w2927) -> (x-y=w2925:dbl)
        n2167 = local read "TEMP"() -> (w2898:dbl)
        n2168 = case shown="True" "Save & Continue" {
          frame False {
          }
          frame True {
            n2169 = local read "Operator ID"() -> (w3426:string)
            n2170 = local read "FILE"() -> (w3432:string)
            n2171 = String Length(string=w3432) -> (length=w3430:i32)
            n2172 = String Length(string=w3426) -> (length=w3427:i32)
            n2173 = Greater?(x=w3430, y=0) -> (0:w3429:bool)
            n2174 = Greater?(x=w3427, y=0) -> (0:w3425:bool)
            n2175 = And(x=w3429, y=w3425) -> (x .and. y?=w3424:bool)
            n2176 = case shown="True" w3424 {
              frame False {
                n2177 = stacked-sequence {
                  frame #0 {
                    n2178 = One Button Dialog(message="Please Enter a File Name and Operator ID to save data !", button name ("OK")="Ok") -> ()  [unwired: 1 out]
                  }
                  frame #1 {
                    n2179 = local write "Save & Continue"(FALSE ("OK Button")) -> ()
                  }
                }
                n2180 = local write "Save & Continue"(FALSE ("OK Button")) -> ()
              }
              frame True {
                n2181 = stacked-sequence {
                  frame #0 {
                    n2182 = call <vilib>:"Application Directory.vi"() -> ("Application Directory"=w3440:path)
                    n2183 = Build Path(base path=w3440, name or relative path="data") -> (appended path=w3439:path)
                    n2184 = local read "FILE"() -> (w3442:string)
                    n2185 = List Folder(path=w3439) -> (folder names=w3438:string[])  [unwired: 3 in, 3 out]
                    n2186 = Equal?(x=w3438, y=w3442) -> (x = y?=w3444:bool[])
                    n2187 = call <vilib>:"Trim Whitespace.vi"("string"=w3442) -> ("trimmed string"=w3437:string)  [unwired: 1 in]
                    n2188 = Or Array Elements(Boolean array=w3444) -> (logical OR=w3443:bool)
                    n2189 = case shown="True" w3443 {
                      tunnel: w3437 -> [_ w3446]
                      frame False {
                      }
                      frame True {
                        w3449 = "_(" ("regular expression")
                        n2190 = Match Pattern(string=w3446, regular expression=w3449) -> (match substring=w3448:string, after substring=w3445:string)  [unwired: 1 in, 2 out]
                        n2191 = Equal?(x=w3448, y=w3449) -> (x = y?=w3447:bool)
                        n2192 = case shown="False" w3447 {
                          tunnel: w3446 -> [w3452 w3462]
                          tunnel: w3445 -> [_ w3464]
                          frame False {
                            n2193 = Concatenate Strings(w3452, "_(" ("regular expression"), "1" ("string"), ")" ("regular expression")) -> (w3450:string)
                            n2194 = local write "FILE"(w3450) -> ()
                          }
                          frame True {
                            n2195 = Decimal String To Number(string=w3464) -> (number=w3463:i32)  [unwired: 2 in, 1 out]
                            n2196 = Search/Split String(string=w3462, search string/char (-)="_(" ("regular expression")) -> (substring before match=w3460:string)  [unwired: 1 in, 2 out]
                            n2197 = Increment(x=w3463) -> (x+1=w3458:i32)
                            n2198 = Number To Decimal String(number=w3458) -> (decimal integer string=w3457:string)  [unwired: 1 in]
                            n2199 = Concatenate Strings(w3460, "_(" ("regular expression"), w3457, ")" ("regular expression")) -> (w3455:string)
                            n2200 = local write "FILE"(w3455) -> ()
                          }
                        }
                      }
                    }
                  }
                  frame #1 {
                    w3475 = 0.0
                    w3477 = cluster{"y":dbl, dbl, "y":dbl}[] [] ("History Data")
                    w3478 = FALSE ("Heater Button")
                    (unwired) ")!" ("string")
                    (unwired) ")" ("string")
                    w3476 = dbl[] [] ("History Data")
                    w3482 = "\r"
                    # "C:\\WinDucom\\Data\\"
                    # "C:\\LAB-IQ-NXT\\data"
                    n2201 = local write "Humidity ( %RH )"(w3475) -> ()
                    n2202 = local write "Frequency ( Hz )"(w3475) -> ()
                    n2203 = local write "speedop"(0.0 ("PIDclk 2")) -> ()
                    n2204 = local write "Set Temp 2"(w3475) -> ()
                    n2205 = local write "AIR TEMP"(w3475) -> ()
                    n2206 = local write "clk"(0.0 ("clk")) -> ()
                    n2207 = local write "Stroke 4"(w3475) -> ()
                    n2208 = local write "Stroke"(w3475) -> ()
                    n2209 = local write "COF 3"(w3475) -> ()
                    n2210 = local write "COF 2"(w3475) -> ()
                    n2211 = local write "TEMP"(w3475) -> ()
                    n2212 = local write "ecr 3"(w3475) -> ()
                    n2213 = local write "FF 3"(w3475) -> ()
                    n2214 = local write "FF 2"(w3475) -> ()
                    n2215 = property on="Humidity ( %RH )" class="WFChart (strict)"("History Data"=w3476) -> ()  [unwired: 2 in, 2 out]
                    n2216 = property on="Coefficient of Friction" class="WFChart (strict)"("History Data"=w3476) -> ()  [unwired: 2 in, 2 out]
                    n2217 = property on="Coefficient of Friction" class="WFChart (strict)"("History Data"=w3476) -> ()  [unwired: 2 in, 2 out]
                    n2218 = property on="Frictional Force ( N )" class="WFChart (strict)"("History Data"=w3476) -> ()  [unwired: 2 in, 2 out]
                    n2219 = property on="Electrical Contact Resistance ( % )" class="WFChart (strict)"("History Data"=w3476) -> ()  [unwired: 2 in, 2 out]
                    n2220 = property on="Electrical Contact Resistance ( % )" class="WFChart (strict)"("History Data"=w3476) -> ()  [unwired: 2 in, 2 out]
                    n2221 = property on="Temperature ( Deg C )" class="WFChart (strict)"("History Data"=w3476) -> ()  [unwired: 2 in, 2 out]
                    n2222 = property on="Frictional Force ( N )" class="WFChart (strict)"("History Data"=w3476) -> ()  [unwired: 2 in, 2 out]
                    n2223 = property on="Coefficient of Friction" class="WFChart (strict)"("History Data"=w3476) -> ()  [unwired: 2 in, 2 out]
                    n2224 = property on="Frictional Force ( N )" class="WFChart (strict)"("History Data"=w3476) -> ()  [unwired: 2 in, 2 out]
                    n2225 = property on="Electrical Contact Resistance ( % )" class="WFChart (strict)"("History Data"=w3476) -> ()  [unwired: 2 in, 2 out]
                    n2226 = property on="Temperature ( Deg C )" class="WFChart (strict)"("History Data"=w3476) -> ()  [unwired: 2 in, 2 out]
                    n2227 = property on="Humidity ( %RH )" class="WFChart (strict)"("History Data"=w3476) -> ()  [unwired: 2 in, 2 out]
                    n2228 = property on="Stroke ( mm )" class="WFChart (strict)"("History Data"=w3477) -> ()  [unwired: 2 in, 2 out]
                    n2229 = property on="Stroke ( mm )" class="WFChart (strict)"("History Data"=w3477) -> ()  [unwired: 2 in, 2 out]
                    n2230 = local write "Humidity"(w3478) -> ()
                    n2231 = local write "Heater Button"(w3478) -> ()
                    n2232 = local read "FILE"() -> (w3471:string)
                    n2233 = local read "NORMAL LOAD"() -> (w3497:dbl)
                    n2234 = call "file check.vi"("file name in"=w3471) -> ("error out"=w3474:errorcluster, "file name out"=w3468:string)  [unwired: 9 in]
                    n2235 = call "FILE PATH CREATION.vi"("error in"=w3474, "FILE NAME :"=w3468) -> ("FILE OUT"=w3467:path)  [unwired: 8 in, 1 out]
                    n2236 = Concatenate Strings(w3468, ".dgf" ("Substring")) -> (w3473:string)
                    n2237 = Concatenate Strings(w3468, ".duf" ("Substring")) -> (w3469:string)
                    n2238 = Multiply(x=w3497, y=1.0) -> (x*y=w3496:dbl)
                    n2239 = Build Path(base path=w3467, name or relative path=w3473) -> (appended path=w3466:path)
                    n2240 = Build Path(base path=w3467, name or relative path=w3469) -> (appended path=w3465:path)
                    n2241 = Number To Fractional String(number=w3496, width (-)=i16 5, precision (6)=i16 2) -> (F-format string=w3505:string)  [unwired: 1 in]
                    n2242 = local read "Fuel Discription :"() -> (w3492:string)
                    n2243 = local read "Batch Ref Num :"() -> (w3480:string)
                    n2244 = Get Date/Time String(date format (0)=enum16{"short", "long", "abbreviated"}."short") -> (date string=w3516:string, time string=w3513:string)  [unwired: 2 in]
                    n2245 = local read "Remarks :"() -> (w3491:string)
                    n2246 = Concatenate Strings("Load :- " ("Substring"), w3505, " N ," ("Substring")) -> (w3504:string)
                    n2247 = local read "String 41"() -> (w3483:string)
                    n2248 = Concatenate Strings(w3492) -> (w3493:string)
                    n2249 = Concatenate Strings(w3480) -> (w3479:string)
                    n2250 = Concatenate Strings("tested by") -> (w3487:string)
                    n2251 = Concatenate Strings("(" ("Substring"), w3516, ")" ("Substring"), w3513) -> (w3485:string)
                    "concatenated string" <- w3485
                    n2252 = Concatenate Strings(w3491, "," ("string")) -> (w3490:string)
                    n2253 = Concatenate Strings("  TIME;      COF;       STROKE;     AIR TEMP;  TEMP;  HUMIDITY;  ECR; PID-OUT; FREQUENCY" ("Substring"), "\r") -> (w3500:string)
                    n2254 = Concatenate Strings(w3483, w3482, "Fuel Discription :-" ("Substring"), w3493, w3482, w3504, w3482, "Batch Ref Num :-" ("Substring"), w3479, w3482, " Remarks :- " ("Substring"), w3490, w3482, " Date :- " ("Substring"), w3485, w3482, "Tested By :-" ("Substring"), w3487) -> (w3498:string)
                    "REMARKS" <- w3498
                    n2255 = call <vilib>:"Write Characters To File.vi"("append to file? (new file:F)"=FALSE, "character string"=w3500, "file path (dialog if empty)"=w3466) -> ()  [unwired: 2 in, 1 out]
                    n2256 = call <vilib>:"Write Characters To File.vi"("append to file? (new file:F)"=FALSE, "character string"=w3498, "file path (dialog if empty)"=w3465) -> ()  [unwired: 2 in, 1 out]
                  }
                  frame #2 {
                    n2257 = local write "Cycles elapsed"(0 ("Cycles elapsed")) -> ()
                    n2258 = local write "cyclecount"(0 ("cyclecount")) -> ()
                    n2259 = local write "Save & Continue"(FALSE ("OK")) -> ()
                    n2260 = local write "autostrtflg"(TRUE ("autostrtflg")) -> ()
                    n2261 = local write "Save"(FALSE ("Save")) -> ()
                    n2262 = Get Date/Time In Seconds() -> (seconds since 1Jan1904=w3522:timestamp)
                    n2263 = To Double Precision Float(number=w3522) -> (double precision float=w3521:dbl)
                    n2264 = local write "acq timer"(w3521) -> ()
                    n2265 = One Button Dialog(message="Please ensure sample is mounted properly and machine is ready in all aspects for testing !", button name ("OK")="Ok") -> ()  [unwired: 1 out]
                  }
                  frame #3 {
                    n2266 = stacked-sequence {
                      frame #0 {
                        n2267 = local write "Main Dashboard Buttons"(T2."Dashboard" ("Main Dashboard Buttons")) -> ()
                        n2268 = local write "Main Tab"(T3."Acquire" ("Main Tab")) -> ()
                      }
                      frame #1 {
                        n2269 = local write "EVENT LOG"("" ("EVENT LOG")) -> ()
                      }
                      frame #2 {
                        n2270 = Wait (ms)(milliseconds to wait=u32 50) -> ()  [unwired: 1 out]
                      }
                      frame #3 {
                        n2271 = disable-structure shown="Disabled" {
                          frame Disabled {
                            n2272 = local read "EVENT LOG"() -> (w3533:string)
                            n2273 = call "Event Log.vi"("Content"="Test Details", "EVENT LOG"=w3533) -> ("EVENT LOG"=w3532:string)  [unwired: 8 in, 1 out]
